vi "Create and Load InverterLUT Dictionary.vi"(8 "error in (no error)":errorcluster, 11 "Main.lvclass":refnum<class "Main.lvclass">) -> (0 "error out":errorcluster, 3 "Main out":refnum<class "Main.lvclass">)   [LabVIEW 2019, in "Main.lvclass"]
doc: "Developed by Kevin Thompson\nkevin@thompsonengineering.net\n\nCopyright 2020\nThompson Engineering, LLC"
uses:
  Main.lvclass
  Main.lvclass/Main.ctl
  Common/DataTypes/Inverter database record v2--cluster.ctl
  Common/DataTypes/inverter info v2--cluster.ctl
  Common/DataTypes/inverter gain range--cluster.ctl
  Common/DataTypes/inverter offset range--cluster.ctl
  Common/DataTypes/Inverter LUT v2--cluster.ctl
  Accessors/Set InverterLUT Dict Ref.vi
  Accessors/Set CurrInverter Record.vi
  Accessors/Get Settings.vi
  <userlib>/_OpenG.lib/file/file.llb/File Exists - Scalar__ogtk.vi
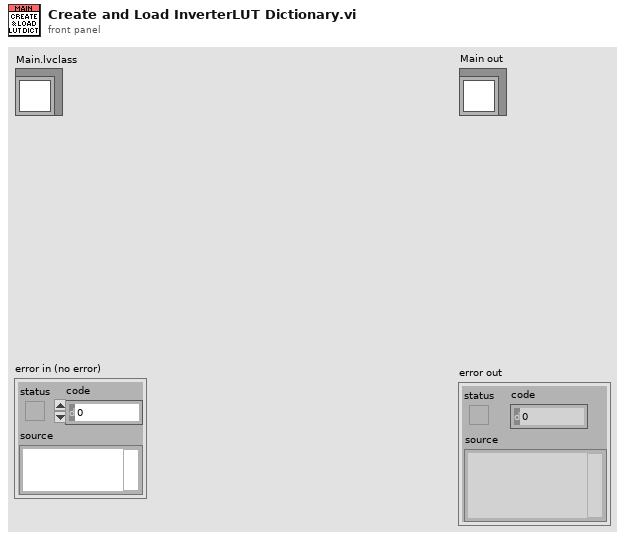
[diagram p1: front panel]
types:
  T1 = typedef "Inverter LUT v2--cluster.ctl" = cluster{"Inverter Records":T2[]}
  T2 = typedef "Inverter database record v2--cluster.ctl" = cluster{"name":string, "last updated":timestamp, "type":string, "inverter Info":T3, "gain range":T4, "offset range":T5, "gain actual":dbl, "offset actual":dbl, "power level":dbl, "minimum current":dbl, "resistance single phase":dbl, "resistance 3 phase":dbl, "set flag":u16}
  T3 = typedef "inverter info v2--cluster.ctl" = cluster{"manufacturer":string, "model":string, "product":string, "serial":string, "power class":string, "year manf":string}
  T4 = typedef "inverter gain range--cluster.ctl" = cluster{"gain max":dbl, "gain min":dbl, "gain increment":dbl}
  T5 = typedef "inverter offset range--cluster.ctl" = cluster{"offset max":dbl, "offset min":dbl, "offset increment":dbl}
  T6 = typedef "Main.lvclass/Settings--cluster.ctl" = cluster{"Simulation":bool, "Signal scaling":T7[], "ESR scaling":T8[], "num readings to average":i32[], "ESR alarm threshhold (%)":i32[], "UseDummyVrms":bool, "Dummy Vrms":dbl, "Inverter Database File":path, "default Inverter (name)":string[], "Minimum Current Threshold ":dbl[], "Sensors Database File":path, "default Sensors (name)":string[]}
  T7 = typedef "Main.lvclass/Gain control.ctl" = cluster{"Iin ripple gain":dbl, "Iout ripple gain":dbl, "Iout 60Hz gain ":dbl, "Vout 60Hz gain ":dbl, "Iin ripple offest":dbl, "Iout ripple offset":dbl, "Iout 60Hz offset":dbl, "Vout 60Hz offset":dbl}
  T8 = typedef "Main.lvclass/ESR scaling--cluster.ctl" = cluster{"Gain":dbl, "Offset":dbl}
  T9 = typedef "TD Dynamic CVT DVR--ref.ctl" = refnum<data-value>
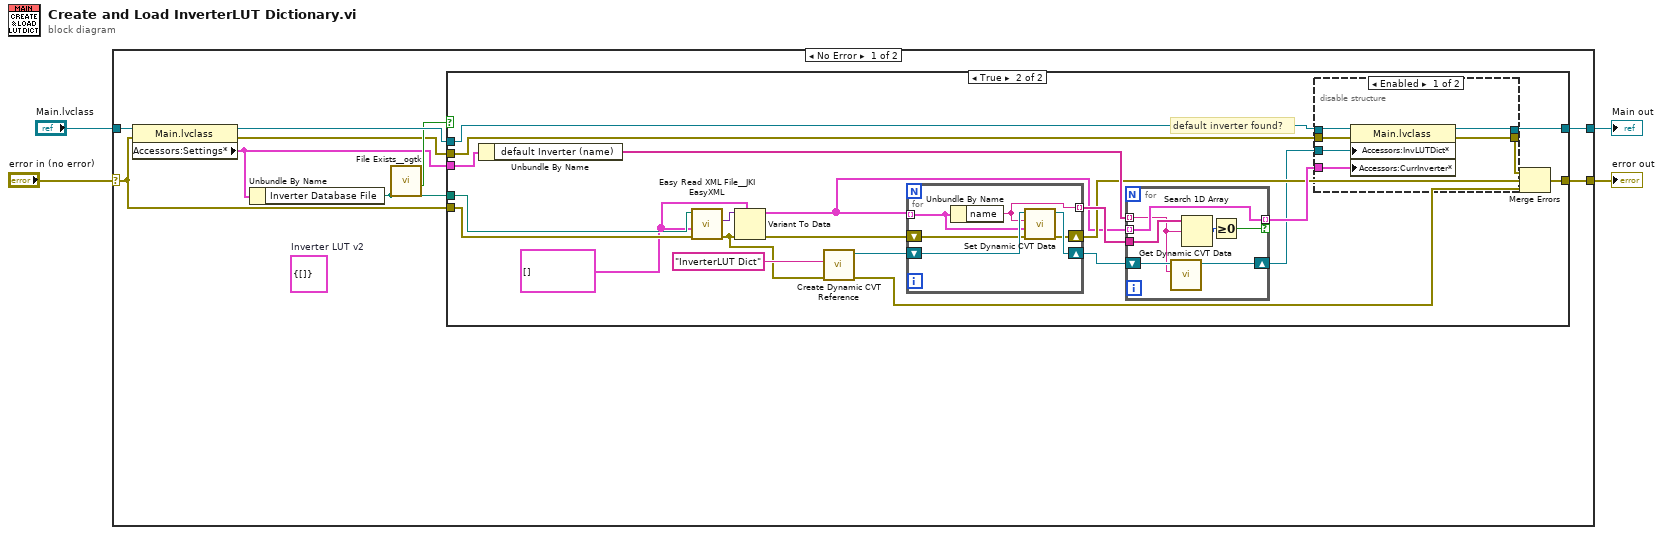
[diagram p0: block diagram]
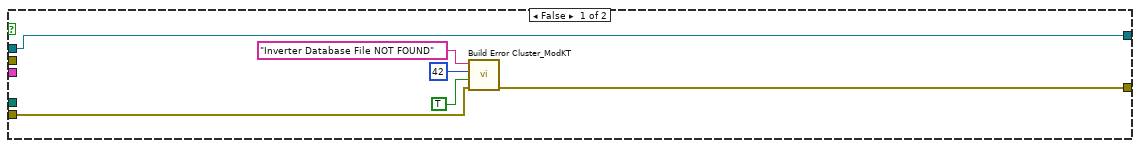
[diagram p2: hidden frame]
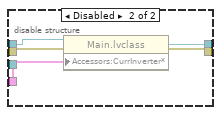
[diagram p3: hidden frame]
diagram:
  n1 = case shown="No Error" "error in (no error)" {
    selector: "error in (no error)" -> [w11 w67]
    tunnel: [w12 w67] -> w1
    tunnel: [w10 w66] -> w2
    tunnel: "Main.lvclass" -> [w13 w66]
    frame No Error {
      (unwired) T1 {"Inverter Records"=[]}  # Inverter LUT v2
      n2 = property class="Main.lvclass"(reference=w13, error in=w11) -> (reference out=w9:refnum<class "Main.lvclass">, error out=w5:errorcluster, "Accessors:Settings*"=w6:T6)
      n3 = Unbundle By Name(w6) -> ("Inverter Database File"=w8:path)
      n4 = call-poly <userlib>:"File Exists__ogtk.vi"("file path"=w8) -> ("exists"=w7:bool)  [unwired: 6 in, 1 out]
      n5 = case shown="True" w7 {
        tunnel: [w18 w29] -> w12
        tunnel: w8 -> [_ w39]
        tunnel: w11 -> [w17 w38]
        tunnel: [w19 w31] -> w10
        tunnel: w9 -> [w19 w37]
        tunnel: w6 -> [_ w32]
        tunnel: w5 -> [_ w30]
        frame False {
          n6 = call <vilib>:"Build Error Cluster_ModKT .vi"("Prepend String (\"\")"="Inverter Database File NOT FOUND" ("Prepend String (\"\")"), "code"=42, "error? (F)"=TRUE, "error in (no error)"=w17) -> ("error out"=w18:errorcluster)  [unwired: 3 in, 1 out]
        }
        frame True {
          w21 = T2[] [] ("Inverter Records")
          # "default inverter found?"
          n7 = Unbundle By Name(w32) -> ("default Inverter (name)"=w26:string[])
          n8 = call <vilib>:"Easy Read XML File__JKI EasyXML.vi"("error in (no error)"=w38, "LabVIEW Data (Type)"=w21, "XML File Path"=w39) -> ("error out"=w36:errorcluster, "LabVIEW Data"=w35:variant)  [unwired: 6 in, 1 out]
          n9 = Variant To Data(error in=w36, type=w21, Variant=w35) -> (data=w22:T2[], error out=w34:errorcluster)
          n10 = call <vilib>:"Create Dynamic CVT Reference.vi"("error in (no error)"=w36, "DictName"="InverterLUT Dict") -> ("error out"=w41:errorcluster, "dCVT DVR out"=w33:T9)  [unwired: 8 in]
          n11 = for {
            tunnel: w22 -> [w61] mode=indexing
            shift-right: [w62] -> w23
            shift-left: w34 -> [w63]
            shift-right: [w64] -> w24
            shift-left: w33 -> [w65]
            tunnel: [w60] -> w27 mode=indexing
            n12 = Unbundle By Name(w61) -> ("name"=w60:string)
            n13 = call <vilib>:"Set Dynamic CVT Data.vi"("error in (no error)"=w63, "value"=w61, "DataName"=w60, "dCVT DVR"=w65) -> ("error out"=w62:errorcluster, "dCVT DVR out"=w64:T9)  [unwired: 5 in, 1 out]
          }
          n14 = for {
            tunnel: w27 -> [w59]
            tunnel: [w56] -> w25 mode=indexing if=w57
            tunnel: w22 -> [w56] mode=indexing
            tunnel: w26 -> [w53] mode=indexing
            shift-right: [w54] -> w20
            shift-left: w24 -> [w55]
            n15 = call <vilib>:"Get Dynamic CVT Data.vi"("DataName"=w53, "dCVT DVR"=w55) -> ("dCVT DVR out"=w54:T9)  [unwired: 6 in, 3 out]
            n16 = Search 1D Array(1D array=w59, element=w53) -> (index of element=w58:i32)  [unwired: 1 in]
            n17 = Greater Or Equal To 0?(x=w58) -> (x >= 0?=w57:bool)
          }
          n18 = disable-structure shown="Enabled" {
            disable-tunnel: w37 -> [w47 w52]
            disable-tunnel: [w46 w48] -> w31
            disable-tunnel: w30 -> [w45 w51]
            disable-tunnel: [w44 w49] -> w28
            disable-tunnel: w25 -> [w43 w50]
            disable-tunnel: w20 -> [w42 _]
            frame Enabled {
              n19 = property class="Main.lvclass"(reference=w47, error in=w45, "Accessors:InvLUTDict*"=w42, "Accessors:CurrInverter*"=w43) -> (reference out=w46:refnum<class "Main.lvclass">, error out=w44:errorcluster)
            }
            frame Disabled {
              n20 = property class="Main.lvclass"(reference=w52, error in=w51, "Accessors:CurrInverter*"=w50) -> (reference out=w48:refnum<class "Main.lvclass">, error out=w49:errorcluster)
            }
          }
          n21 = Merge Errors(w28, w23, w41) -> (w29:errorcluster)
        }
      }
    }
    frame Error {
    }
  }
  "error out" <- w1
  "Main out" <- w2
